vi "Set Bulk Stream Size.vi"(7 "SlaveID":u8, 8 "error in (no error)":errorcluster, 11 ".NET Refnum in":refnum<k24>) -> (0 "error out":errorcluster, 3 ".NET Refnum out":refnum<k24>)   [LabVIEW 2013]
uses:
  C:/Users/User/Desktop/Modbus Demo/DLL/Modbus.dll
  DLL/Modbus.dll
panel:
  out "Vib_dat":u16[](array[numeric])
  out "Length Check":i16
  in  "Stream Size (9)":i16=9
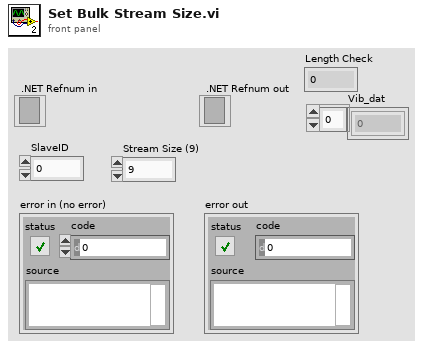
[diagram p1: front panel]
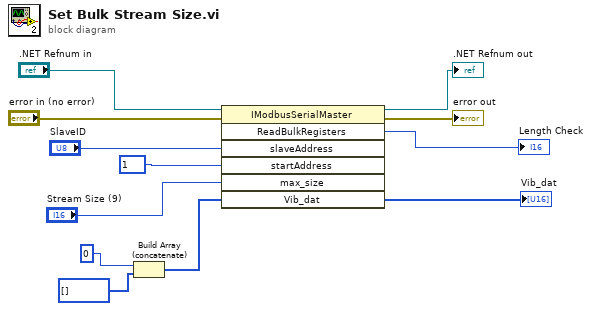
[diagram p0: block diagram]
diagram:
  n1 = Build Array (concatenate)(u16 0, u16[] [] ("Vib_dat")) -> (w1:u16[])
  n2 = invoke class="IModbusSerialMaster" method="ReadBulkRegisters"(reference=".NET Refnum in", error in="error in (no error)", "slaveAddress"="SlaveID", "startAddress"=u16 1, "max_size"="Stream Size (9)", "Vib_dat"=w1) -> (reference out=→".NET Refnum out":refnum<k24>, error out=→"error out":errorcluster, "ReadBulkRegisters"=→"Length Check":i16, "Vib_dat"=→"Vib_dat":u16[])  [unwired: 1 in, 3 out]
